vi "GetCtlRef_Wrap.vi"(8 "error in (no error)":errorcluster, 10 "Control Label":string, 11 "CtlLookup In":T1) -> (0 "error out":errorcluster, 2 "CtlRef Out":refnum<vi>, 3 "CtlLookup Out":T1)   [LabVIEW 2020]
doc: "This is the base of the polymorphic VI \"GetControlRef\" \n\nThis is a General Helper VI.\n\nThis will search the incoming \"Ref Cluster\" for the Control Label string. If it finds it, it will output the reference If it does not, it will create an error -8000 with the control name"
uses:
  TypeDefs/CtlLookup.ctl
  CtlReferences.lvclass
  Error_CtlNotFound.vi
  <vilib>/Utility/error.llb/Error Cluster From Error Code.vi
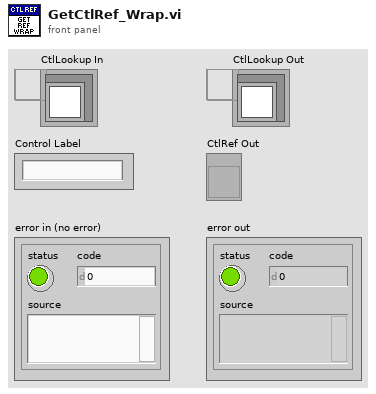
[diagram p1: front panel]
types:
  T1 = typedef "CtlReferences.lvlib/CtlReferences.lvclass/CtlLookup.ctl" = refnum<data-value>
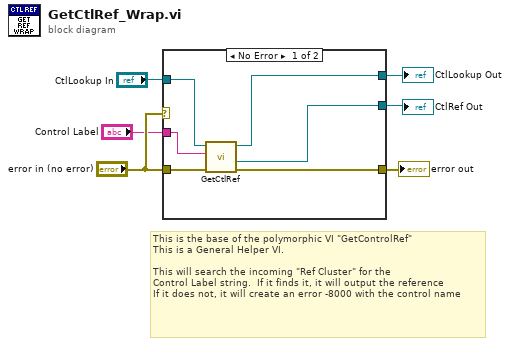
[diagram p0: block diagram]
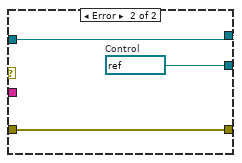
[diagram p2: hidden frame]
diagram:
  # "This is the base of the polymorphic VI \"GetControlRef\"\nThis is a General Helper VI.\n\nThis will search the incoming \"Ref Cluster\" for the \nControl Label string.  If it finds it, it will output the reference\nIf it does not, it will create an error -8000 with the control name"
  n1 = case shown="No Error" "error in (no error)" {
    tunnel: [w9 w15] -> w6
    tunnel: "error in (no error)" -> [w8 w15]
    tunnel: "CtlLookup In" -> [w12 w14]
    tunnel: [w10 w14] -> w3
    tunnel: [w7 w13] -> w2
    tunnel: "Control Label" -> [w11 _]
    frame No Error {
      n2 = call "GetCtlRef.vi"("Error in"=w8, "CtlName In"=w11, "CtlLookup In"=w12) -> ("error out"=w9:errorcluster, "CtlRef"=w7:refnum<vi>, "CtlLookup Out"=w10:T1)  [unwired: 5 in, 1 out]
    }
    frame Error {
      w13 = refnum<vi> refnum  # Control
    }
  }
  "error out" <- w6
  "CtlLookup Out" <- w3
  "CtlRef Out" <- w2
